vi "GetHeaderValue.vi"(1 "Server Frame":T1, 3 "Header Name":string, 5 "error in":errorcluster) -> (15 "Value":string, 17 "Found?":bool, 19 "error out":errorcluster)   [LabVIEW 2017, in "STOMP.lvclass"]
uses:
  STOMP.lvclass
  Typedefs/Type_ServerFrame.ctl
  Typedefs/Type_ServerFrameType.ctl
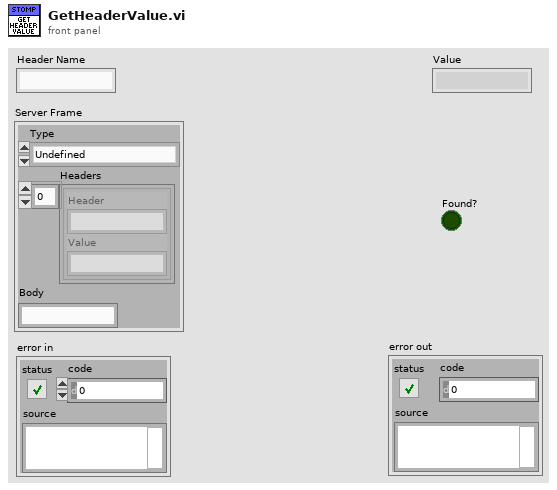
[diagram p1: front panel]
types:
  T1 = typedef "STOMP.lvclass/Type_ServerFrame.ctl" = cluster{"Type":T2, "Headers":cluster{"Header":string, "Value":string}[], "Body":string}
  T2 = typedef "STOMP.lvclass/Type_ServerFrameType.ctl" = enum16{"Undefined", "MESSAGE", "CONNECTED", "RECEIPT", "ERROR"}
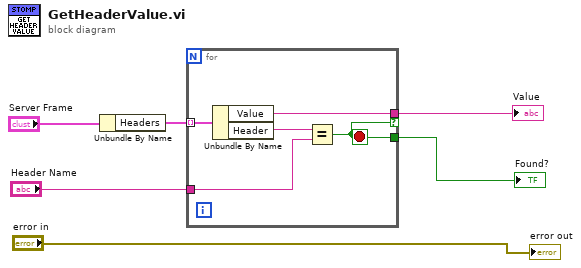
[diagram p0: block diagram]
diagram:
  n1 = Unbundle By Name("Server Frame") -> ("Headers"=w5:cluster{"Header":string, "Value":string}[])
  n2 = for {
    tunnel: w5 -> [w11] mode=indexing
    tunnel: "Header Name" -> [w9]
    tunnel: [w8] -> w3 if=w7
    tunnel: [w7] -> w2
    stop <- w7 stop-if-true
    n3 = Unbundle By Name(w11) -> ("Value"=w8:string, "Header"=w10:string)
    n4 = Equal?(x=w10, y=w9) -> (x = y?=w7:bool)
  }
  "Value" <- w3
  "Found?" <- w2
  "error out" <- "error in"
